vi "Get Log File Type.vi"(8 "error in (no error)":errorcluster, 11 "Log File in":refnum<class "Log File.lvclass">) -> (0 "error out":errorcluster, 2 "Log File Type":T1, 3 "Log File out":refnum<class "Log File.lvclass">)   [LabVIEW 2015, in "Log File.lvclass"]
uses:
  Log File.lvclass
  Log File Type.ctl
  Log File.lvclass/Log File.ctl
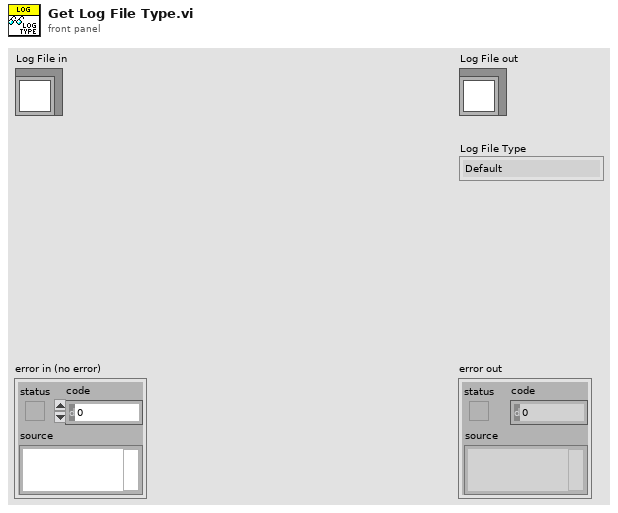
[diagram p1: front panel]
types:
  T1 = typedef "Log File.lvclass/Log File Type.ctl" = enum16{"Default", "TDMS", "Text"}
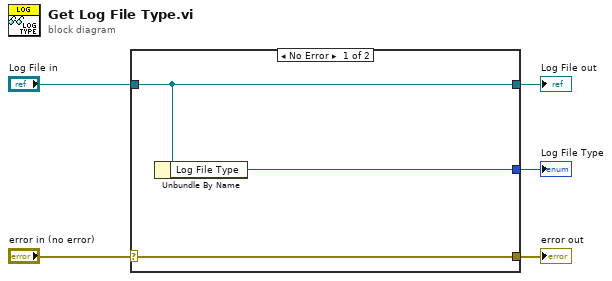
[diagram p0: block diagram]
diagram:
  n1 = case shown="No Error" "error in (no error)" {
    selector: "error in (no error)" -> [w8 w9]
    tunnel: [w8 w9] -> w4
    tunnel: [w7 w10] -> w2
    tunnel: "Log File in" -> [w7 w10]
    tunnel: [w6 _] -> w1
    frame No Error {
      n2 = Unbundle By Name(w7) -> ("Log File Type"=w6:T1)
    }
    frame Error {
    }
  }
  "error out" <- w4
  "Log File out" <- w2
  "Log File Type" <- w1
